vi "Read output.vi"(8 "error in (no error)":errorcluster, 10 "Bytes to read":u32=10 min=1, 11 "Read handle":u64) -> (0 "error out":errorcluster, 3 "String out":string)   [LabVIEW 2012, in "LightPipes.lvlib"]
uses:
  LightPipes.lvlib
  kernel32.dll
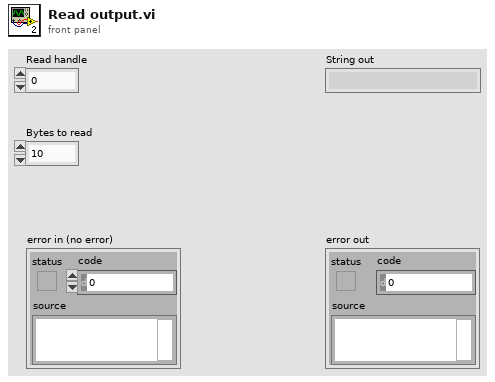
[diagram p1: front panel]
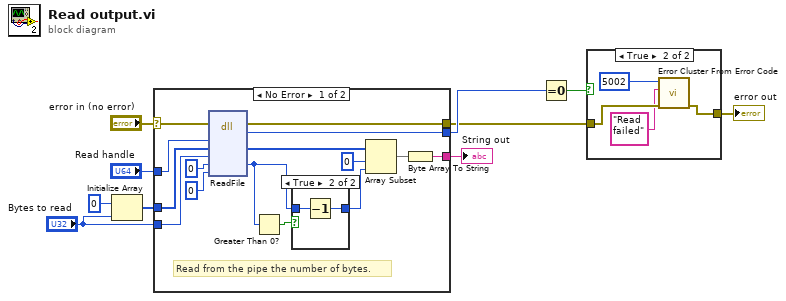
[diagram p0: block diagram]
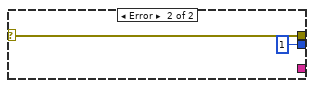
[diagram p4: hidden frame]
diagram:
  n1 = Initialize Array(u8 0 ("element"), "Bytes to read") -> (w9:u8[])
  n2 = case shown="No Error" "error in (no error)" {
    selector: "error in (no error)" -> [w18 w30]
    tunnel: w9 -> [w25 _]
    tunnel: "Bytes to read" -> [w24 _]
    tunnel: "Read handle" -> [w17 _]
    tunnel: [w13 _] -> w5
    tunnel: [w12 1 ("BOOL")] -> w4
    tunnel: [w11 w30] -> w3
    frame No Error {
      # "Read from the pipe the number of bytes."
      n3 = dll-call lib="kernel32.dll" fn="ReadFile"(error in=w18, "hFile"=w17, "lpBuffer"=w25, "nNumberOfBytesToRead"=w24, "lpNumberOfBytesRead"=u32 0, "lpOverlapped"=u64 0) -> (error out=w11:errorcluster, "BOOL"=w12:i32, "lpBuffer"=w21:u8[], "lpNumberOfBytesRead"=w15:u32)  [unwired: 5 in, 1 out]
      n4 = Greater Than 0?(x=w15) -> (x > 0?=w14:bool)
      n5 = case shown="True" w14 {
        tunnel: w15 -> [w26 w28]
        tunnel: [w26 w27] -> w16
        frame False {
        }
        frame True {
          n6 = Decrement(x=w28) -> (x-1=w27:u32)
        }
      }
      n7 = Array Subset(array=w21, index=0, length=w16) -> (w19:u8[])
      n8 = Byte Array To String(unsigned byte array=w19) -> (string=w13:string)
    }
    frame Error {
    }
  }
  "String out" <- w5
  n9 = Equal To 0?(x=w4) -> (x = 0?=w1:bool)
  n10 = case shown="True" w1 {
    tunnel: w3 -> [w31 w35]
    tunnel: [w31 w34] -> w2
    frame False {
    }
    frame True {
      n11 = call <vilib>:"Error Cluster From Error Code.vi"("error in (no error)"=w35, "error message (\"\")"="Read  failed" ("error message (\"\")"), "error code (0)"=5002) -> ("error out"=w34:errorcluster)  [unwired: 6 in]
    }
  }
  "error out" <- w2
